vi "set_internal_files.vi"(8 "error in (no error)":errorcluster, 11 "pulse_gen_and_detect_p2p in":refnum<class "pulse_gen_and_detect_p2p.lvclass">) -> (0 "error out":errorcluster, 3 "pulse_gen_and_detect_p2p out":refnum<class "pulse_gen_and_detect_p2p.lvclass">)   [LabVIEW 2021, in "pulse_gen_and_detect_p2p.lvclass"]
uses:
  pulse_gen_and_detect_p2p.lvclass
  classes/device_type/device_type.lvclass
  pulse_gen_and_detect_p2p.lvclass/pulse_gen_and_detect_p2p.ctl
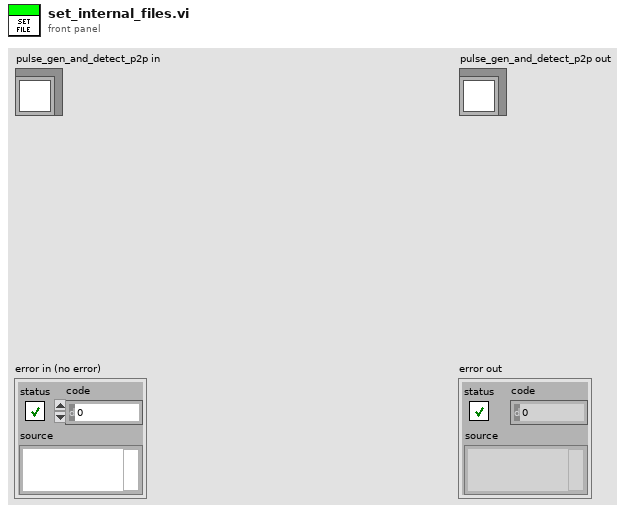
[diagram p1: front panel]
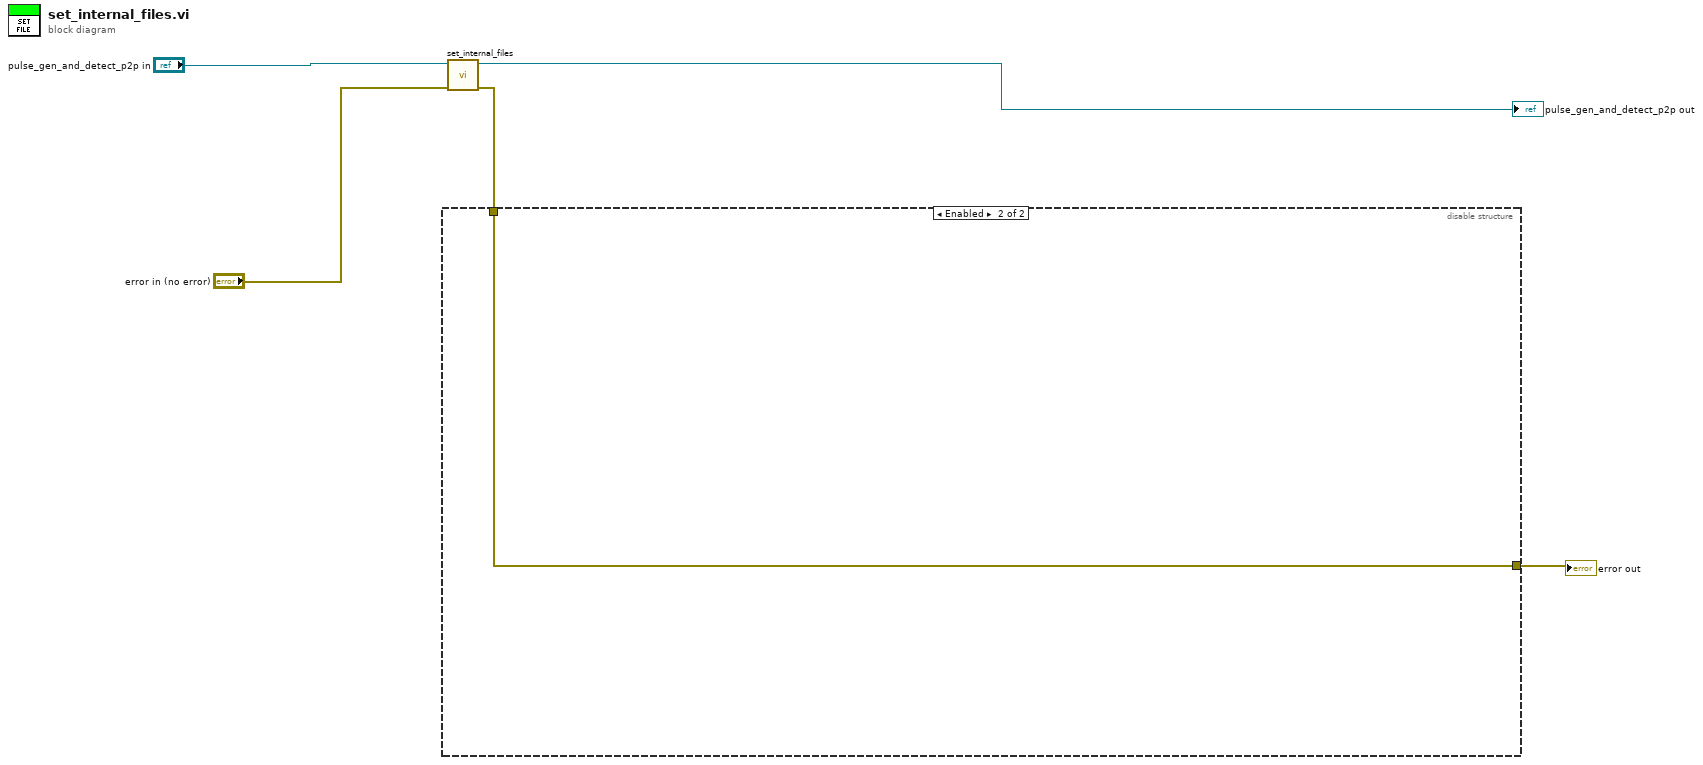
[diagram p0: block diagram]
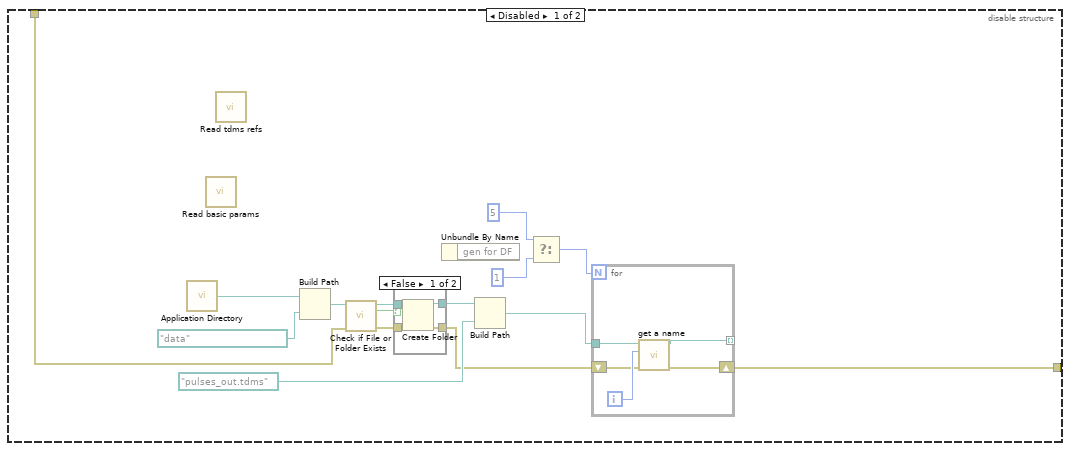
[diagram p2: hidden frame]
diagram:
  n1 = call-parent "set_internal_files.vi"("error in (no error)"="error in (no error)", "device_type in"="pulse_gen_and_detect_p2p in") -> ("error out"=w2:errorcluster, "device_type out"=→"pulse_gen_and_detect_p2p out":refnum<class "pulse_gen_and_detect_p2p.lvclass">)  [unwired: 8 in]
  n2 = disable-structure shown="Enabled" {
    disable-tunnel: w2 -> [w7 w32]
    disable-tunnel: [w6 w32] -> w1
    frame Disabled {
      n3 = call <vilib>:"Application Directory.vi"() -> ("Application Directory"=w16:path)
      n4 = call-dynamic "Read basic params.vi"() -> ()  [unwired: 14 in, 6 out]
      n5 = call-dynamic "Read tdms refs.vi"() -> ()  [unwired: 9 in, 3 out]
      n6 = Build Path(base path=w16, name or relative path=path "data") -> (appended path=w13:path)
      n7 = call <vilib>:"Check if File or Folder Exists.vi"("error in (no error)"=w7, "path"=w13) -> ("error out"=w10:errorcluster, "file or folder exists?"=w8:bool, "dup path"=w12:path)  [unwired: 7 in]
      n8 = case shown="False" w8 {
        tunnel: w12 -> [w24 w26]
        tunnel: [w23 w26] -> w11
        tunnel: w10 -> [w22 w25]
        tunnel: [w21 w25] -> w9
        frame False {
          n9 = Create Folder(path (use dialog)=w24, error in=w22) -> (created path=w23:path, error out=w21:errorcluster)  [unwired: 1 in, 1 out]
        }
        frame True {
        }
      }
      n10 = Unbundle By Name() -> ()  [unwired: 1 in, 1 out]
      n11 = Build Path(base path=w11, name or relative path=path "pulses_out.tdms") -> (appended path=w14:path)
      n12 = Select(t=5, f=1) -> (s? t:f=w20:i32)  [unwired: 1 in]
      n13 = for {
        N: w20 -> [_]
        tunnel: w14 -> [w31]
        shift-right: [w28] -> w6
        shift-left: w9 -> [w29]
        tunnel: [w27] -> _ mode=indexing
        i -> [w30]
        n14 = call "get a name.vi"("error constant"=w29, "Numeric"=w30, "Bitfile path"=w31) -> ("error constant 2"=w28:errorcluster, "Path"=w27:path)  [unwired: 7 in]
      }
    }
    frame Enabled {
    }
  }
  "error out" <- w1
